vi "Calc Combined Metric v2.vi"() -> ()   [LabVIEW 2014]
panel:
  out "Isign":dbl=-1.0
  in  "Sign Look Up":i32[][](array[numeric])=[[2, -1], [3, -1], [4, -1], [5, -1], [6, -1], [7, 1], [8, 1], [9, -1], [10, -1], [11, -1], [22, 1], [37, 1]]
  in  "k":dbl=0.01
  out "b":dbl=1.0
  in  "a":dbl=1.0
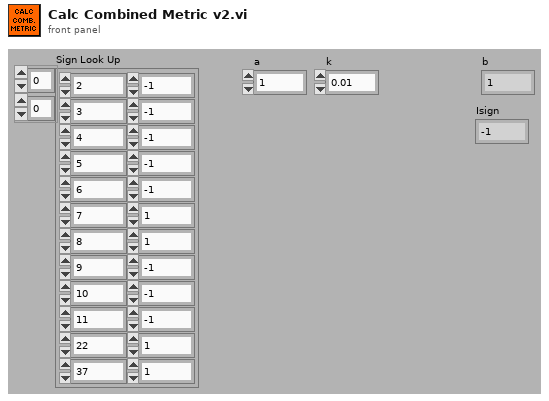
[diagram p1: front panel]
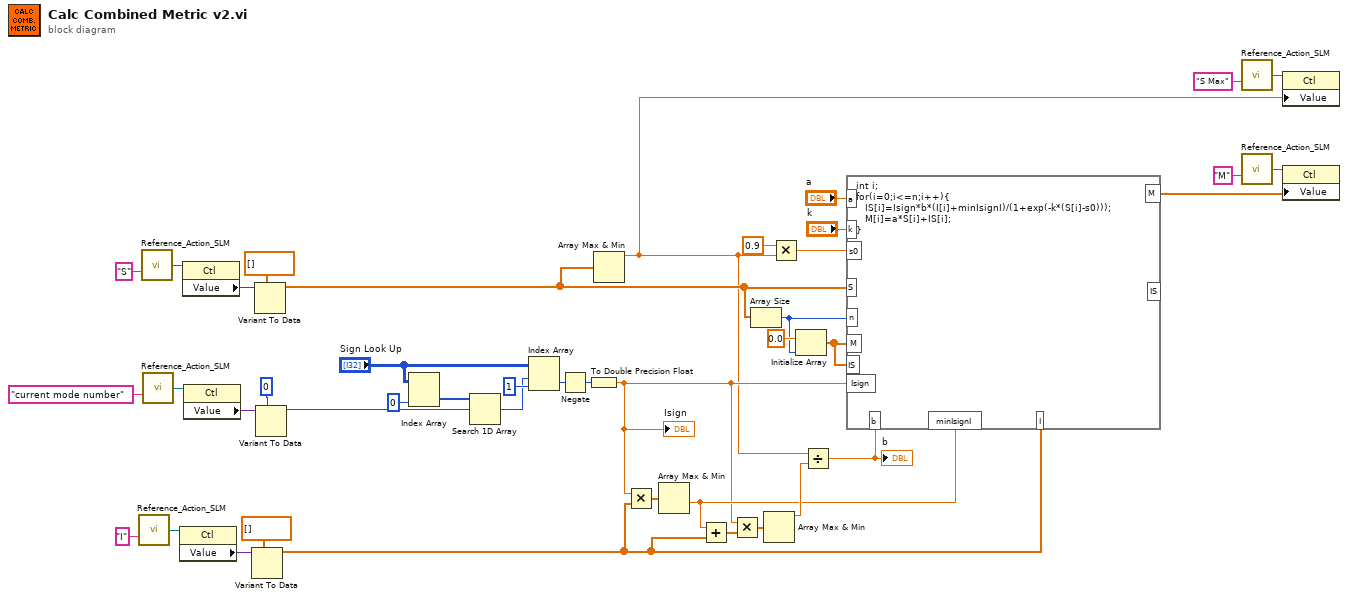
[diagram p0: block diagram]
diagram:
  n1 = call "Reference_Action_SLM.vi"("Control Name"="I") -> ("Ref OUT"=w17:refnum<vi>)  [unwired: 12 in, 2 out]
  n2 = call "Reference_Action_SLM.vi"("Control Name"="S") -> ("Ref OUT"=w12:refnum<vi>)  [unwired: 12 in, 2 out]
  n3 = call "Reference_Action_SLM.vi"("Control Name"="current mode number") -> ("Ref OUT"=w20:refnum<vi>)  [unwired: 12 in, 2 out]
  n4 = property class="Ctl"(reference=w17) -> ("Value"=w16:variant)  [unwired: 1 in, 2 out]
  n5 = property class="Ctl"(reference=w12) -> ("Value"=w11:variant)  [unwired: 1 in, 2 out]
  n6 = property class="Ctl"(reference=w20) -> ("Value"=w19:variant)  [unwired: 1 in, 2 out]
  n7 = Variant To Data(type=dbl[] [] ("Ab Corr VI.I"), Variant=w16) -> (data=w14:dbl[])  [unwired: 1 in, 1 out]
  n8 = Variant To Data(type=dbl[] [] ("Ab Corr VI.I"), Variant=w11) -> (data=w9:dbl[])  [unwired: 1 in, 1 out]
  n9 = Variant To Data(type=0 ("disabled index (col)"), Variant=w19) -> (data=w2:i32)  [unwired: 1 in, 1 out]
  n10 = Index Array(array="Sign Look Up", index (col)=0 ("disabled index (col)")) -> (element=w28:i32[])  [unwired: 1 in]
  n11 = Search 1D Array(1D array=w28, element=w2) -> (index of element=w25:i32)  [unwired: 1 out]
  n12 = Index Array(array="Sign Look Up", index (row)=w25, index (col)=1 ("disabled index (col)")) -> (element=w24:i32)
  n13 = Negate(x=w24) -> (-x=w23:i32)
  n14 = To Double Precision Float(number=w23) -> (double precision float=w22:dbl)
  "Isign" <- w22
  n15 = Array Max & Min(array=w9) -> (max value=w1:dbl)  [unwired: 3 out]
  n16 = Multiply(x=w22, y=w14) -> (x*y=w34:dbl[])
  n17 = Array Max & Min(array=w34) -> (min value=w31:dbl)  [unwired: 3 out]
  n18 = Add(x=w31, y=w14) -> (x+y=w33:dbl[])
  n19 = Multiply(x=w22, y=w33) -> (x*y=w32:dbl[])
  n20 = Array Size(array=w9) -> (size(s)=w37:i32)
  n21 = Array Max & Min(array=w32) -> (max value=w36:dbl)  [unwired: 3 out]
  n22 = Multiply(x=0.9, y=w1) -> (x*y=w30:dbl)
  n23 = Initialize Array(0.0 ("element"), w37) -> (w40:dbl[])
  n24 = Divide(x=w1, y=w36) -> (x/y=w35:dbl)
  "b" <- w35
  n25 = formula code="int i;\nfor(i=0;i<=n;i++){\n   IS[i]=Isign*b*(I[i]+minIsignI)/(1+exp(-k*(S[i]-s0)));\n   M[i]=a*S[i]+IS[i];\n}"("a"="a", "k"="k", "s0"=w30, "S"=w9, "I"=w14, "n"=w37, "IS"=w40, "M"=w40, "b"=w35, "Isign"=w22, "minIsignI"=w31) -> ("M"=w4:dbl[])  [unwired: 1 out]
  n26 = call "Reference_Action_SLM.vi"("Control Name"="S Max") -> ("Ref OUT"=w7:refnum<vi>)  [unwired: 12 in, 2 out]
  n27 = call "Reference_Action_SLM.vi"("Control Name"="M") -> ("Ref OUT"=w5:refnum<vi>)  [unwired: 12 in, 2 out]
  n28 = property class="Ctl"(reference=w7, "Value"=w1) -> ()  [unwired: 1 in, 2 out]
  n29 = property class="Ctl"(reference=w5, "Value"=w4) -> ()  [unwired: 1 in, 2 out]
